vi "pulse.vi"(4 "error in":errorcluster, 5 "dwell after":u32, 6 "time on":u32, 7 "lines 2":tag) -> (0 "error out":errorcluster)   [LabVIEW 2012]
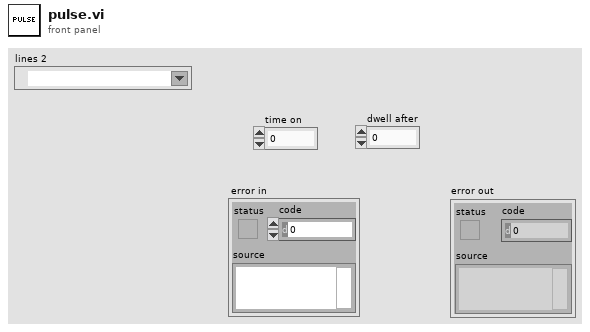
[diagram p1: front panel]
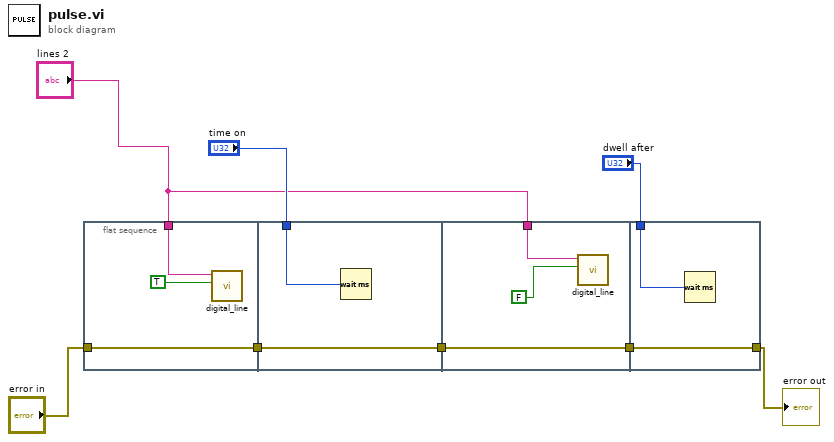
[diagram p0: block diagram]
diagram:
  n1 = flat-sequence {
    tunnel: "error in" -> [w11]
    tunnel: [w11] -> w6
    tunnel: "lines 2" -> [w9]
    tunnel: "time on" -> [w13]
    tunnel: w6 -> [w12]
    tunnel: [w12] -> w5
    tunnel: w5 -> [w16]
    tunnel: "lines 2" -> [w15]
    tunnel: [w16] -> w4
    tunnel: [w18] -> w3
    tunnel: w4 -> [w18]
    tunnel: "dwell after" -> [w17]
    frame #0 {
      n2 = call "digital_line.vi"("Boolean"=TRUE ("NewVal"), "lines"=w9) -> ()  [unwired: 5 in, 1 out]
    }
    frame #1 {
      n3 = Wait (ms)(milliseconds to wait=w13) -> ()  [unwired: 1 out]
    }
    frame #2 {
      n4 = call "digital_line.vi"("Boolean"=FALSE ("NewVal"), "lines"=w15) -> ()  [unwired: 5 in, 1 out]
    }
    frame #3 {
      n5 = Wait (ms)(milliseconds to wait=w17) -> ()  [unwired: 1 out]
    }
  }
  "error out" <- w3
